vi "readU8.vi"(8 "error in (no error)":errorcluster, 11 "IU8Control in":refnum<class "IU8Control.lvclass">) -> (0 "error out":errorcluster, 2 "Data":u8, 3 "IU8Control out":refnum<class "IU8Control.lvclass">)   [LabVIEW 2016, in "RTFPGA.lvlib" / "IU8Control.lvclass"]
uses:
  IU8Control.lvclass
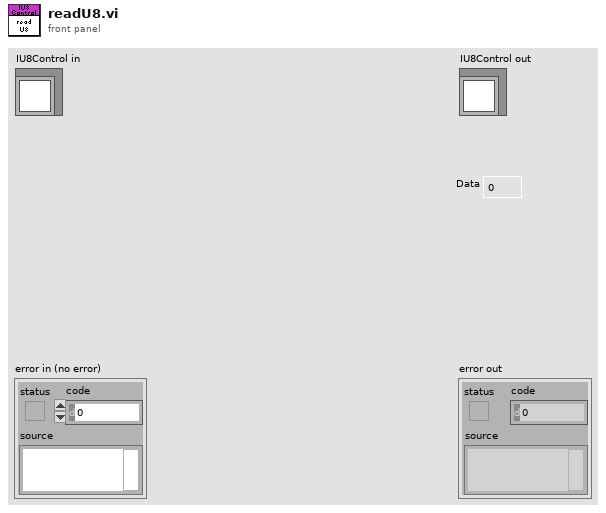
[diagram p1: front panel]
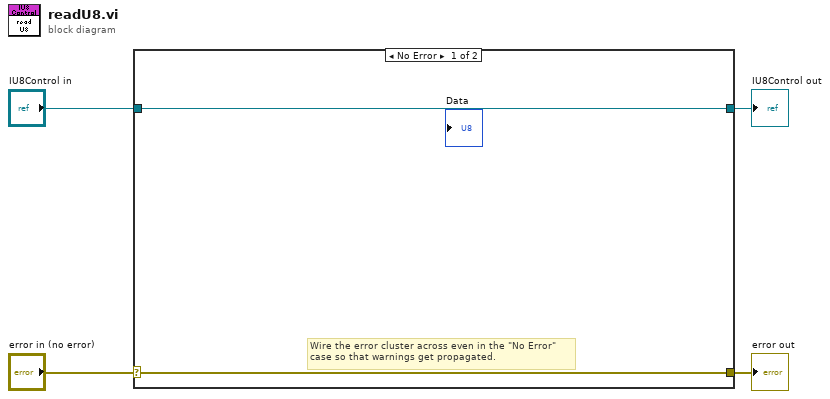
[diagram p0: block diagram]
diagram:
  n1 = case shown="No Error" "error in (no error)" {
    selector: "error in (no error)" -> [w5 w8]
    tunnel: [w5 w8] -> w3
    tunnel: [w6 w7] -> w1
    tunnel: "IU8Control in" -> [w6 w7]
    frame No Error {
      # "Wire the error cluster across even in the \"No Error\"\ncase so that warnings get propagated."
    }
    frame Error {
    }
  }
  "error out" <- w3
  "IU8Control out" <- w1
